vi "TeamLeader.vi"(10 "TL?":bool, 11 "Enum in":refnum<vi>) -> ()   [LabVIEW 2020]
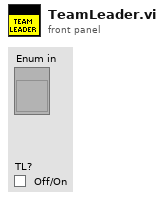
[diagram p1: front panel]
types:
  T1 = enum8{"Enabled", "Disabled", "Disabled and Grayed Out"}
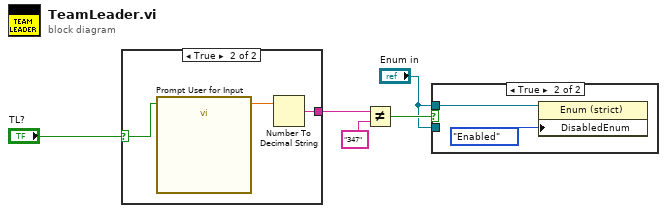
[diagram p0: block diagram]
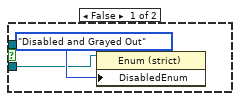
[diagram p2: hidden frame]
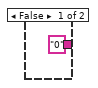
[diagram p3: hidden frame]
diagram:
  n1 = case shown="True" "TL?" {
    selector: "TL?" -> [_ w7]
    tunnel: ["0" w8] -> w2
    frame False {
    }
    frame True {
      n2 = call "Prompt User for Input"("Enable"=w7) -> ("Code :"=w9:dbl)  [unwired: 16 in, 2 out]
      n3 = Number To Decimal String(number=w9) -> (decimal integer string=w8:string)  [unwired: 1 in]
    }
  }
  n4 = Not Equal?(x=w2, y="347") -> (x != y?=w4:bool)
  n5 = case shown="True" w4 {
    tunnel: "Enum in" -> [w10 _]
    tunnel: "Enum in" -> [_ w12]
    frame False {
      n6 = property on="Property Node" class="Enum (strict)"(reference=w10, "DisabledEnum"=T1."Disabled and Grayed Out" ("Disabled")) -> ()  [unwired: 1 in, 2 out]
    }
    frame True {
      n7 = property on="Property Node" class="Enum (strict)"(reference=w12, "DisabledEnum"=T1."Enabled" ("Disabled")) -> ()  [unwired: 1 in, 2 out]
    }
  }
